vi "ScriptedAutonomous.vi"   [LabVIEW 2014]
uses:
  Robot Global Data.vi
types:
  T1 = typedef "commandCluster.ctl" = cluster{"Step ID":i32, "Command Type":i32, "Drive X":dbl, "Drive Y":dbl, "Heading":dbl, "Max Exec. Time":u32, "Jump Type":i32, "Jump To":i32, "Jump Condition":i32, "Coast":i32, "Speed":dbl, "Init ID":i32, "Init Type":i32, "Pk":dbl, "Ik":dbl, "Dk":dbl}
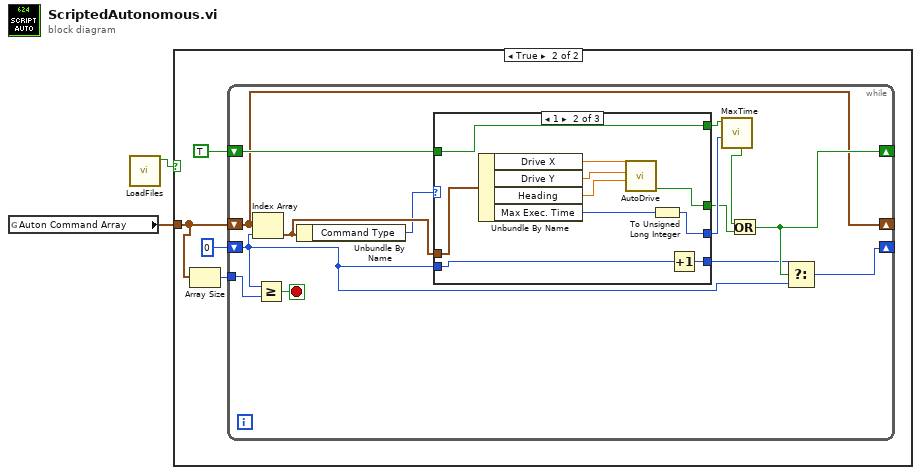
[diagram p0: block diagram]
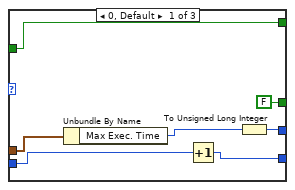
[diagram p3: hidden frame]
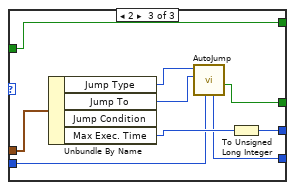
[diagram p4: hidden frame]
diagram:
  n1 = global read "Robot Global Data.vi" "Auton Command Array"() -> (w1:T1[])
  n2 = call "LoadFiles.vi"() -> ("Done?"=w2:bool)  [unwired: 11 in]
  n3 = case shown="True" w2 {
    tunnel: w1 -> [_ w6]
    frame False {
    }
    frame True {
      n4 = Array Size(array=w6) -> (size(s)=w3:i32)
      n5 = while {
        shift-right: [w8] -> _
        shift-left: w6 -> [w8]
        shift-right: [w13] -> _
        shift-left: 0 -> [w12]
        shift-right: [w20] -> _
        shift-left: TRUE -> [w14]
        tunnel: w3 -> [w10]
        stop <- w11 stop-if-true
        n6 = Index Array(array=w8, index=w12) -> (element=w9:T1)
        n7 = Greater Or Equal?(x=w12, y=w10) -> (x >= y?=w11:bool)
        n8 = Unbundle By Name(w9) -> ("Command Type"=w7:i32)
        n9 = case shown="1" w7 {
          tunnel: [w22 w34 w46] -> w19
          tunnel: w9 -> [w27 w37 w42]
          tunnel: w12 -> [w26 w36 w39]
          tunnel: [w23 w35 w40] -> w18
          tunnel: [FALSE w29 w41] -> w17
          tunnel: [w25 w28 w38] -> w15
          tunnel: w14 -> [w25 w28 w38]
          frame 0, Default {
            n10 = Unbundle By Name(w27) -> ("Max Exec. Time"=w21:u32)
            n11 = Increment(x=w26) -> (x+1=w23:i32)
            n12 = To Unsigned Long Integer(number=w21) -> (unsigned 32bit integer=w22:u32)
          }
          frame 1 {
            n13 = Unbundle By Name(w37) -> ("Drive X"=w33:dbl, "Drive Y"=w32:dbl, "Heading"=w31:dbl, "Max Exec. Time"=w30:u32)
            n14 = call "AutoDrive.vi"("Heading"=w31, "Drive Y"=w32, "Drive X"=w33) -> ("Done?"=w29:bool)  [unwired: 8 in]
            n15 = To Unsigned Long Integer(number=w30) -> (unsigned 32bit integer=w34:u32)
            n16 = Increment(x=w36) -> (x+1=w35:i32)
          }
          frame 2 {
            n17 = Unbundle By Name(w42) -> ("Jump Type"=w45:i32, "Jump To"=w44:i32, "Max Exec. Time"=w43:u32)  [unwired: 1 out]
            n18 = call "AutoJump.vi"("Current Index"=w39, "Goto"=w44, "Type"=w45) -> ("Done?"=w41:bool, "New Index"=w40:i32)  [unwired: 7 in]
            n19 = To Unsigned Long Integer(number=w43) -> (unsigned 32bit integer=w46:u32)
          }
        }
        n20 = call "MaxTime.vi"("maxTime"=w19, "Reset?"=w15) -> ("Finished?"=w16:bool)  [unwired: 9 in]
        n21 = Or(x=w16, y=w17) -> (x .or. y?=w20:bool)
        n22 = Select(t=w18, s=w20, f=w12) -> (s? t:f=w13:i32)
      }
    }
  }
